vi "Preview Start.vi"(8 "error in":errorcluster, 9 "分辨率":string, 10 "preview path":u8) -> (0 "error out":errorcluster, 2 "return":i32)   [LabVIEW 2016]
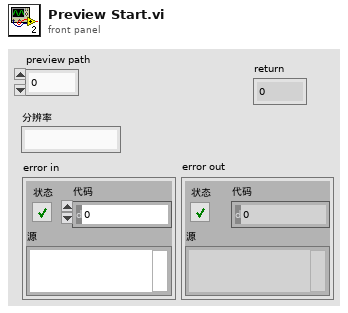
[diagram p1: front panel]
types:
  T1 = cluster{"byCmdType":u8, "bySubCmd":u8, "byPara":u8, "byAddr_h":u8, "byAddr_l":u8, "byAddr_ll":u8, "byLen_h":u8, "byLen_l":u8}
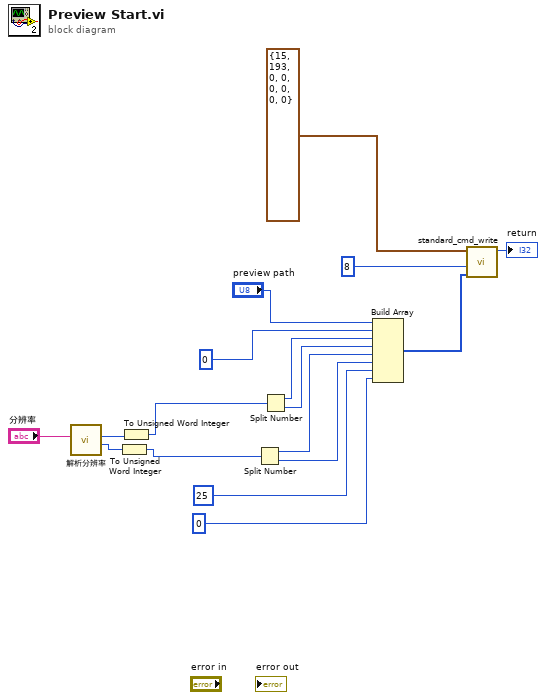
[diagram p0: block diagram]
diagram:
  n1 = call "解析分辨率.vi"("分辨率"="分辨率") -> ("number 2"=w4:i32, "number"=w5:i32)  [unwired: 9 in]
  n2 = To Unsigned Word Integer(number=w4) -> (unsigned 16bit integer=w2:u16)
  n3 = To Unsigned Word Integer(number=w5) -> (unsigned 16bit integer=w3:u16)
  n4 = Split Number(x=w2) -> (hi(x)=w12:u8, lo(x)=w11:u8)
  n5 = Split Number(x=w3) -> (hi(x)=w14:u8, lo(x)=w13:u8)
  n6 = Build Array("preview path", u8 0, w14, w13, w12, w11, u8 25, u8 0) -> (w8:u8[])
  n7 = call "standard_cmd_write.vi"("data"=w8, "dwLen"=u32 8, "cmd_std_header_t"=T1 {"byCmdType"=15, "bySubCmd"=193, "byPara"=0, "byAddr_h"=0, "byAddr_l"=0, "byAddr_ll"=0, "byLen_h"=0, "byLen_l"=0}) -> ("return"=→"return":i32)  [unwired: 7 in, 1 out]
